vi "反馈节点.vi"() -> ()   [LabVIEW 2010]
panel:
  out "输出前次循环的值":dbl
  out "输出本次循环的值":dbl
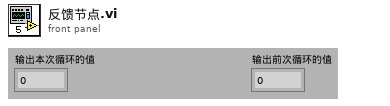
[diagram p1: front panel]
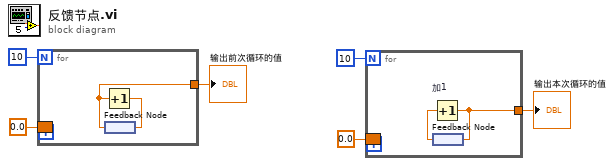
[diagram p0: block diagram]
diagram:
  n1 = for {
    N: 10 -> [_]
    tunnel: [w8] -> w1
    border: 0.0 -> [_]
    n2 = feedback #1() -> (w8:dbl)
    n3 = Increment(x=w8) -> (x+1=w7:dbl)
    n4 = feedback-in #1(w7) -> ()
  }
  "输出前次循环的值" <- w1
  n5 = for {
    N: 10 -> [_]
    tunnel: [w9] -> w3
    border: 0.0 -> [_]
    n6 = feedback #2() -> (w10:dbl)
    n7 = Increment "加1"(x=w10) -> (x+1=w9:dbl)
    n8 = feedback-in #2(w9) -> ()
  }
  "输出本次循环的值" <- w3
